vi "SD-Read From XML File.vi"   [LabVIEW 2020]
doc: "Reads and parses tags from a LabVIEW XML file. When you place this VI on the block diagram, the polymorphic VI selector is visible. Use this selector to choose which polymorphic instance to use. All XML data must follow the standard LabVIEW XML schema."
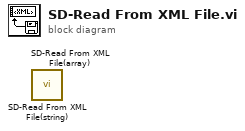
[diagram p0: block diagram]
diagram:
  n1 = call "SD-Read From XML File(string).vi"() -> ()  [unwired: 9 in, 3 out]
  n2 = call "SD-Read From XML File(array).vi"() -> ()  [unwired: 9 in, 3 out]
